vi "Harmonic Distortion Analyzer N Chan.vi"(6 "advanced search":T4={"approx freq. (optional)"=-1.0, "search (+/- % of Fsampl.)"=5.0} {"search (+/- % of Fsampl.)" format="%0.2p"; "approx freq. (optional)" format="%0.2p"}, 7 "stop search at Nyquist":bool=TRUE, 8 "error in (no error)":errorcluster, 9 "highest harmonic":i32=19, 10 "export mode":T2(ring), 11 "signals in":waveform(dbl)[](array[waveform])) -> (0 "error out":errorcluster, 1 "components levels":cluster{"components level":dbl[]}[](array[cluster]) {"components level" format="%.2p"}, 2 "THD":dbl[](array[numeric]) format="%.2p", 3 "detected fundamental frequencies":dbl[](array[numeric]) format="%.2p", 4 "measurements info":T3(array[cluster]) {"uncertainty" format="%0.2p"}, 5 "exported signals":T1(array[cluster]) {"exported spectrum (dB)"."dB Spectrum (Hann)" format="%.2p"; "exported spectrum (dB)"."df" format="%.2p"; "exported spectrum (dB)"."f0" format="%.2p"})   [LabVIEW 2020, in "NI_MAPro.lvlib"]
doc: "Takes a signal in and performs a full harmonic analysis, including measuring the fundamental frequency tone and harmonics, and returning the fundamental frequency, all harmonic amplitude levels, and the total harmonic distortion (THD). Wire data to the <B>signal in</B> input to determine the polymorphic instance to use or manually select the instance."
uses:
  NI_MAPro.lvlib
  NI_MABase.lvlib
panel:
  # "Harmonic Distortion\nAnalyzer"
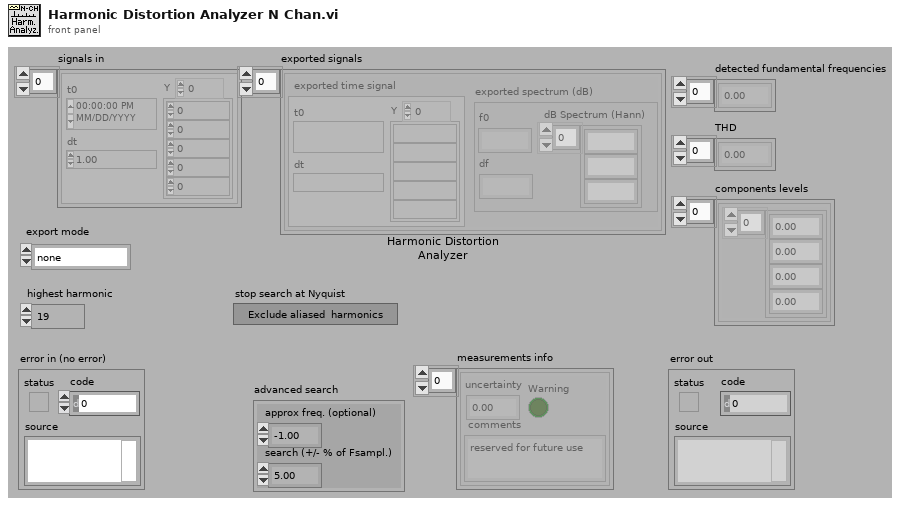
[diagram p1: front panel]
types:
  T1 = cluster{"exported time signal":waveform(dbl), "exported spectrum (dB)":cluster{"f0":dbl, "df":dbl, "dB Spectrum (Hann)":dbl[]}}[]
  T2 = enum16{"none", "input signal", "fundamental signal", "residual signal", "harmonics only", "noise and spurs"}
  T3 = cluster{"uncertainty":dbl, "Warning":bool, "comments":string}[]
  T4 = cluster{"approx freq. (optional)":dbl, "search (+/- % of Fsampl.)":dbl}
  T5 = cluster{"uncertainty":dbl, "Warning":bool, "comments":string}
  T6 = cluster{"exported time signal":waveform(dbl), "exported spectrum (dB)":cluster{"f0":dbl, "df":dbl, "dB Spectrum (Hann)":dbl[]}}
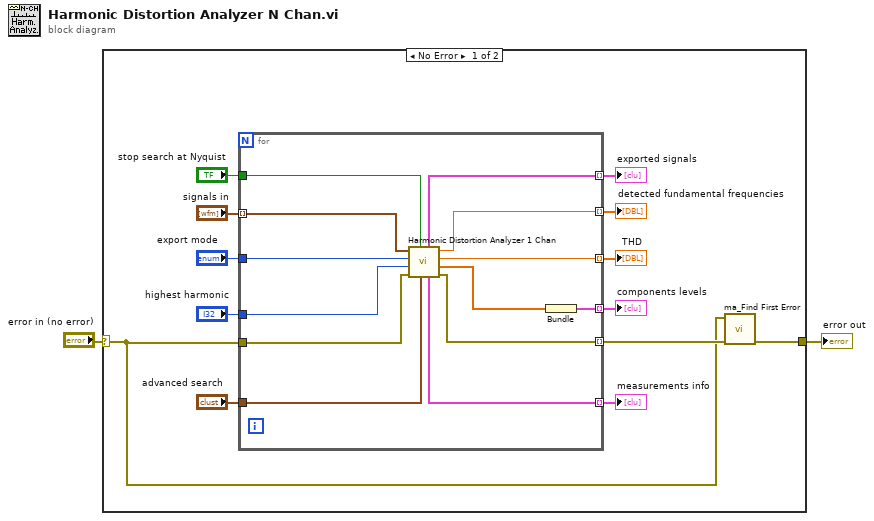
[diagram p0: block diagram]
diagram:
  n1 = case shown="No Error" "error in (no error)" {
    selector: "error in (no error)" -> [w5 w29]
    tunnel: [w8 w29] -> w2
    frame No Error {
      n2 = for {
        tunnel: [w19] -> w15 mode=indexing
        tunnel: [w18] -> w14 mode=indexing
        tunnel: [w22] -> w13 mode=indexing
        tunnel: "signals in" -> [w27] mode=indexing
        tunnel: [w17] -> w11 mode=indexing
        tunnel: [w16] -> w10 mode=indexing
        tunnel: w5 -> [w25]
        tunnel: [w21] -> w9 mode=indexing
        tunnel: "stop search at Nyquist" -> [w28]
        tunnel: "advanced search" -> [w26]
        tunnel: "highest harmonic" -> [w24]
        tunnel: "export mode" -> [w23]
        n3 = call "Harmonic Distortion Analyzer 1 Chan.vi"("advanced search"=w26, "stop search at Nyquist"=w28, "error in (no error)"=w25, "highest harmonic"=w24, "export mode"=w23, "signal in"=w27) -> ("error out"=w21:errorcluster, "components level"=w20:dbl[], "THD"=w18:dbl, "detected fundamental frequency"=w16:dbl, "measurement info"=w22:T5, "exported signals"=w17:T6)
        n4 = Bundle("components level"=w20) -> (w19:cluster{"components level":dbl[]})  [unwired: 1 in]
      }
      "detected fundamental frequencies" <- w10
      "THD" <- w14
      "components levels" <- w15
      "measurements info" <- w13
      "exported signals" <- w11
      n5 = call "ma_Find First Error.vi"("error array in"=w9, "error in 1 (no error)"=w5) -> ("error out"=w8:errorcluster)  [unwired: 2 in, 3 out]
    }
    frame Error {
    }
  }
  "error out" <- w2
